vi "Continuous Pulse Generator at 1KHz.vi"() -> ()   [LabVIEW 2019, in "Part of Main VIs.lvlib" / "Tachometer Library.lvlib"]
uses:
  <vilib>/Platform/TimedLoop/XDataNode/timing_clust.ctl
  <vilib>/Platform/TimedLoop/XDataNode/nitl_modes.ctl
  <vilib>/Platform/TimedLoop/XDataNode/wakeup.ctl
  <vilib>/numeric/Random Number (Range) DBL.vi
  <vilib>/DAQmx/create/channels.llb/DAQmx Create Channel (CO-Pulse Generation-Time).vi
  <vilib>/DAQmx/configure/timing.llb/DAQmx Timing (Implicit).vi
  <vilib>/Platform/TimedLoop/XDataNode/XDataNode.xnode
  Tachometer Library.lvlib
  <resource>/objmgr/daqmx.rc
  <vilib>/Platform/TimedLoop/XDataNode/XDNodeRunTimeDep.lvlib
panel:
  out "TeleMetry History":string
  out "x-y 3":dbl
  out "Pulse Period 2":dbl
  out "Pulse Frequency 2":dbl
  out "Numeric 2":i32
  out "Numeric 3":i32
  out "Pulse LowTime":dbl
  out "Pulse HighTime":dbl
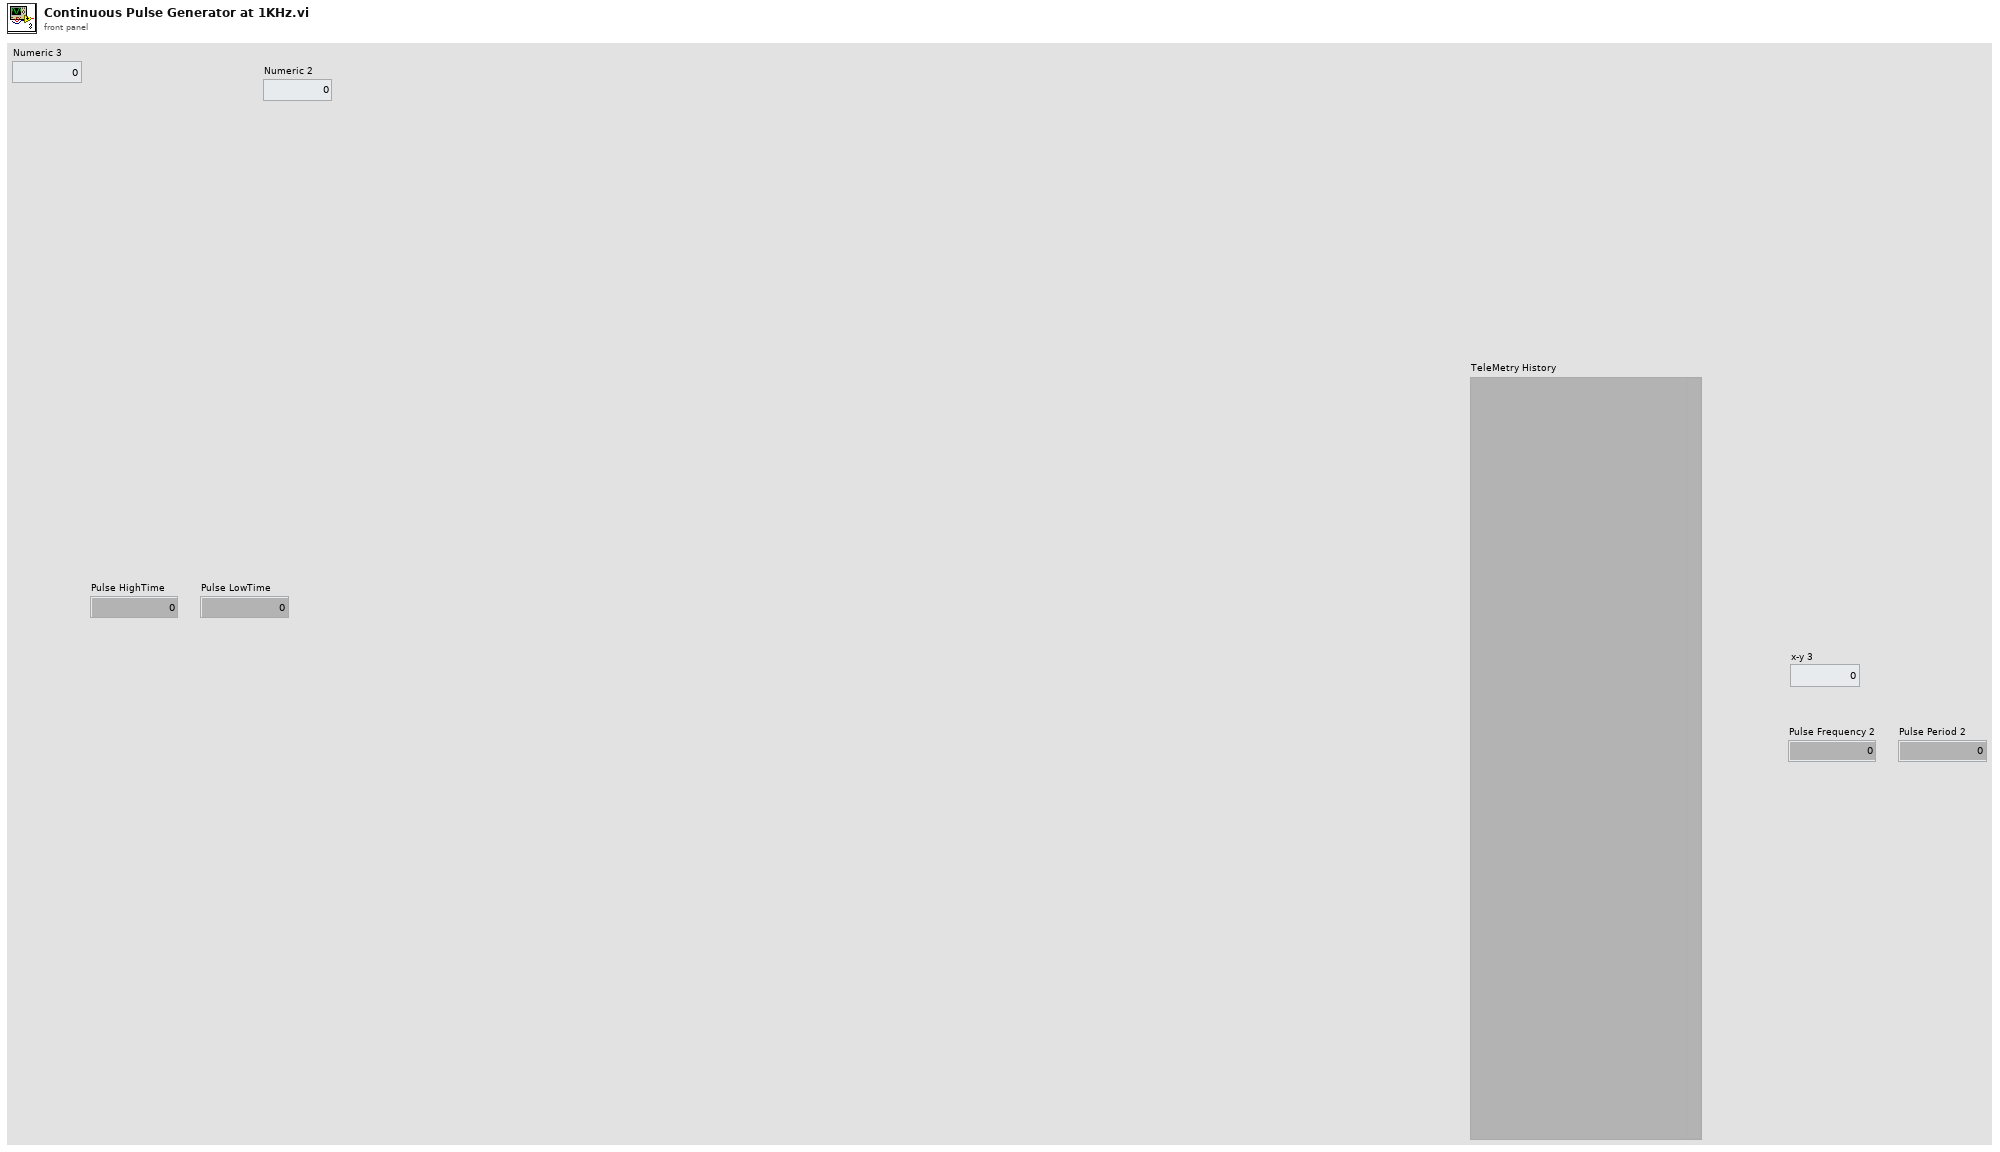
[diagram p1: front panel]
types:
  T1 = typedef "XDNodeRunTimeDep.lvlib/timing_clust.ctl" = cluster{"Expected End [f-1]":u64, "Actual End [f-1]":u64, "Finished Late? [f-1]":bool, "Expected End [i-1]":u64, "Actual End [i-1]":u64, "Finished Late? [i-1]":bool, "Expected Start [i]":u64, "Actual Start [i]":u64, "Expected Start [f]":u64, "Actual Start [f]":u64, "Source Name":string, "Structure Name":string, "Period":i64, "Deadline":i64, "Offset":i64, "Start":i64, "Priority":i32, "Timeout":i32, "Mode":T2, "Wakeup Reason":T3, "Error":errorcluster, "Source Type":string, "Secondary Source Type":string, "Global End Time":u64, "Global Start Time":u64, "Frame Duration":u64, "Iteration Duration":u64, "Assigned CPU":i32, "I/O Scan Engine Mode":u32}
  T2 = typedef "XDNodeRunTimeDep.lvlib/nitl_modes.ctl" = enum32{"No Change", "Process missed periods, maintain original phase", "Discard missed periods, maintain original phase", "Process missed periods, ignore original phase", "Discard missed periods, ignore original phase"}
  T3 = typedef "XDNodeRunTimeDep.lvlib/wakeup.ctl" = enum32{"Normal", "Aborted", "Asynchronous wakeup", "Timing source error", "Timed loop error", "Timeout"}
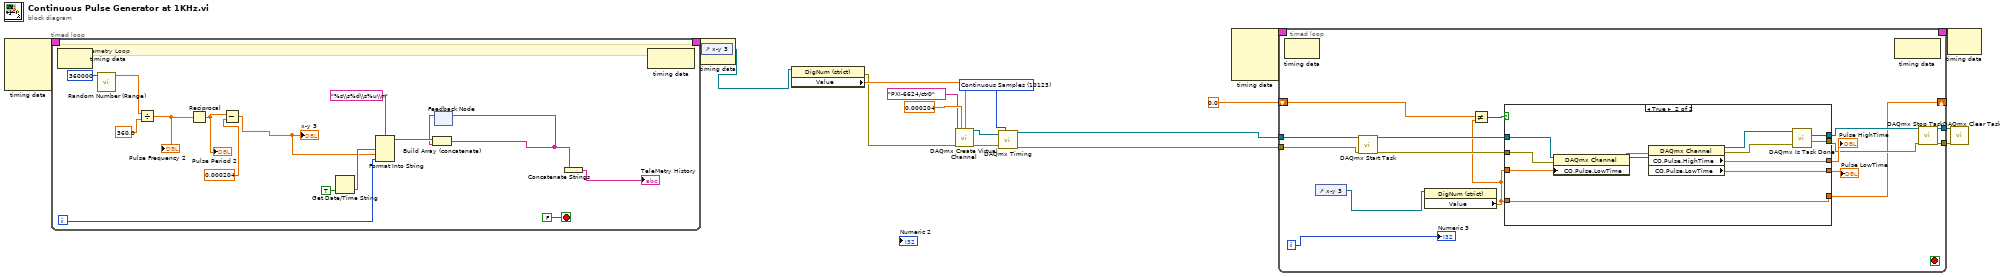
[diagram p0: block diagram]
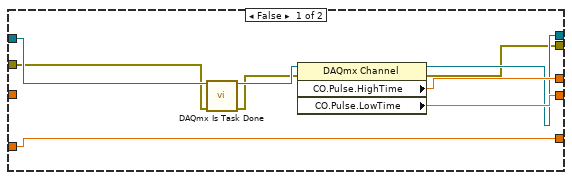
[diagram p2: hidden frame]
diagram:
  w5 = 10123 items=["Finite Samples"=10178, "Continuous Samples"=10123, "Hardware Timed Single Point"=12522] ("sample mode")
  n1 = node-c288() -> (w2:T1)  [unwired: 4 in]
  n2 = timed-loop {
    timing: w2 -> [_]
    timing-out: [_] -> w1
    i -> [w18]
    stop <- FALSE stop-if-true
    # "Part of Telemetry Loop"
    n3 = node-c288() -> ()  [unwired: 1 in, 1 out]
    n4 = call-poly <vilib>:"Random Number (Range).vi"("upper bound (100)"=u64 360000) -> ("number"=w33:dbl)  [unwired: 10 in]
    n5 = Divide(x=w33, y=360.0) -> (x/y=w31:dbl)
    "Pulse Frequency 2" <- w31
    n6 = Reciprocal(x=w31) -> (1/x=w32:dbl)
    "Pulse Period 2" <- w32
    n7 = Subtract(x=w32, y=0.000204 ("high time")) -> (x-y=w19:dbl)
    "x-y 3" <- w19
    n8 = Get Date/Time String(want seconds? (F)=TRUE) -> (time string=w21:string)  [unwired: 2 in, 1 out]
    n9 = Format Into String(format string="%s\\s%d\\s%u\\n", w21, w19, w18) -> (resulting string=w25:string)  [unwired: 2 in, 1 out]
    n10 = feedback #1() -> (w23:string[])  [unwired: 1 in]
    n11 = Build Array (concatenate)(w25, w23) -> (w22:string[])
    n12 = feedback-in #1(w22) -> ()
    n13 = Concatenate Strings(w22) -> (→"TeleMetry History":string)
    n14 = node-c288() -> ()  [unwired: 1 in, 1 out]
  }
  n15 = node-c288(w1) -> ()  [unwired: 1 out]
  n16 = control-ref of="x-y 3"() -> (w4:refnum<vi>)
  n17 = property class="DigNum (strict)"(reference=w4) -> (error out=w10:errorcluster, "Value"=w11:dbl)  [unwired: 1 in, 1 out]
  n18 = call-poly <vilib>:"DAQmx Create Virtual Channel.vi"("high time"=0.000204, "low time"=w11, "counter"=tag "PXI-6624/ctr0", "error in"=w10) -> ("task out"=w16:refnum<k21>, "error out"=w15:errorcluster)  [unwired: 10 in]
  n19 = call-poly <vilib>:"DAQmx Timing.vi"("task/channels in"=w16, "sample mode"=w5, "error in"=w15) -> ("task out"=w7:refnum<k21>, "error out"=w6:errorcluster)  [unwired: 11 in]
  n20 = node-c288() -> (w9:T1)  [unwired: 4 in]
  n21 = timed-loop {
    timing: w9 -> [_]
    timing-out: [_] -> w8
    tunnel: [w50] -> w12
    tunnel: [w51] -> w13
    tunnel: w7 -> [w42]
    tunnel: w6 -> [w41]
    shift-right: [w36] -> _
    shift-left: 0.0 ("element") -> [w38]
    i -> [w40]
    stop <- _ stop-if-true
    n22 = node-c288() -> ()  [unwired: 1 in, 1 out]
    n23 = control-ref of="x-y 3"() -> (w39:refnum<vi>)
    n24 = call <vilib>:"DAQmx Start Task.vi"("task/channels in"=w42, "error in"=w41) -> ("task out"=w46:refnum<k21>, "error out"=w45:errorcluster)  [unwired: 12 in]
    n25 = property class="DigNum (strict)"(reference=w39) -> ("Value"=w37:dbl)  [unwired: 1 in, 2 out]
    n26 = Not Equal?(x=w38, y=w37) -> (x != y?=w49:bool)
    n27 = case shown="True" w49 {
      tunnel: [w56 w72] -> w44
      tunnel: [w55 w71] -> w43
      tunnel: [w58 w68] -> w48
      tunnel: [w57 w67] -> w47
      tunnel: w46 -> [w54 w64]
      tunnel: w45 -> [w53 w63]
      tunnel: w37 -> [_ w62]
      tunnel: [w52 w61] -> w36
      tunnel: w37 -> [w52 w61]
      frame False {
        n28 = call <vilib>:"DAQmx Is Task Done.vi"("task/channels in"=w54, "error in"=w53) -> ("task out"=w60:refnum<k21>, "error out"=w59:errorcluster)  [unwired: 11 in, 1 out]
        n29 = property class="DAQmx Channel"(reference=w60, error in=w59) -> (reference out=w56:refnum<k21>, error out=w55:errorcluster, "CO.Pulse.HighTime"=w58:dbl, "CO.Pulse.LowTime"=w57:dbl)
      }
      frame True {
        n30 = property class="DAQmx Channel"(reference=w64, error in=w63, "CO.Pulse.LowTime"=w62) -> (reference out=w70:refnum<k21>, error out=w69:errorcluster)
        n31 = property class="DAQmx Channel"(reference=w70, error in=w69) -> (reference out=w66:refnum<k21>, error out=w65:errorcluster, "CO.Pulse.HighTime"=w68:dbl, "CO.Pulse.LowTime"=w67:dbl)
        n32 = call <vilib>:"DAQmx Is Task Done.vi"("task/channels in"=w66, "error in"=w65) -> ("task out"=w72:refnum<k21>, "error out"=w71:errorcluster)  [unwired: 11 in, 1 out]
      }
    }
    "Pulse HighTime" <- w48
    "Pulse LowTime" <- w47
    n33 = node-c288() -> ()  [unwired: 1 in, 1 out]
    n34 = call <vilib>:"DAQmx Stop Task.vi"("task/channels in"=w44, "error in"=w43) -> ("task out"=w50:refnum<k21>, "error out"=w51:errorcluster)  [unwired: 12 in]
    "Numeric 3" <- w40
  }
  n35 = node-c288(w8) -> ()  [unwired: 1 out]
  n36 = call <vilib>:"DAQmx Clear Task.vi"("task in"=w12, "error in"=w13) -> ()  [unwired: 13 in, 1 out]
